vi "Close RT data queue.vi"(11 "RT Queues":T1) -> ()   [LabVIEW 2018]
uses:
  Type Defs/Queues cluster.ctl
  ICL-LabVIEW_General/Message Scheduler/message scheduler.lvclass
types:
  T1 = typedef "Queues cluster.ctl" = cluster{"RT Message":refnum<queue>, "RT Comms":refnum<queue>, "RT Data":refnum<queue>, "RT FIFO":refnum<queue>, "message scheduler":refnum<class "message scheduler.lvclass">}
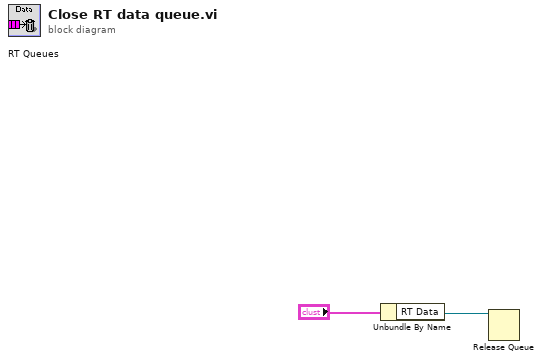
[diagram p0: block diagram]
diagram:
  n1 = Unbundle By Name("RT Queues") -> ("RT Data"=w2:refnum<queue>)
  n2 = Release Queue(queue=w2) -> ()  [unwired: 2 in, 3 out]
